vi "Get_Rise_Fall_Time.vi"(10 "Transition_Points":i32[](array[numeric]), 11 "dt":dbl) -> (2 "Fall_Time (s)":dbl, 3 "Rise_Time (s)":dbl)   [LabVIEW 2023]
doc: "This VI Get the rise and fall time when transition points and dt were given in."
uses:
  <vilib>/gmath/NI_Gmath.lvlib
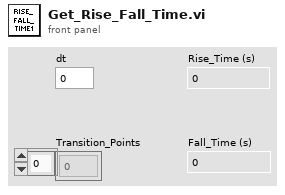
[diagram p1: front panel]
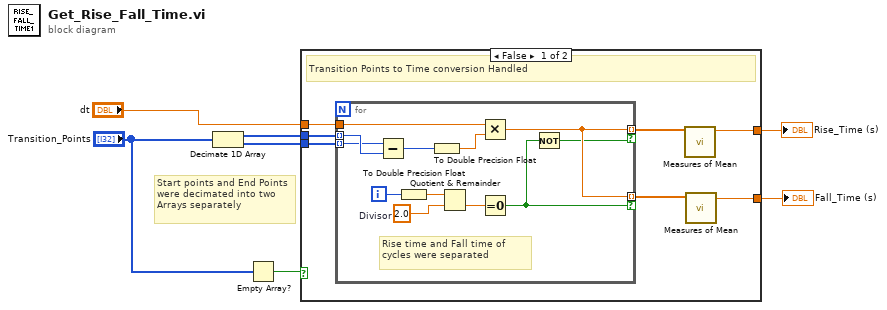
[diagram p0: block diagram]
diagram:
  # "Start points and End Points were decimated into two Arrays separately"
  n1 = Decimate 1D Array("Transition_Points") -> (w3:i32[], w4:i32[])
  n2 = Empty Array?(array="Transition_Points") -> (empty?=w1:bool)
  n3 = case shown="False" w1 {
    tunnel: [w14 _] -> w7
    tunnel: [w12 _] -> w6
    tunnel: "dt" -> [w10 _]
    tunnel: w4 -> [w9 _]
    tunnel: w3 -> [w8 _]
    frame False {
      # "Transition Points to Time conversion Handled"
      n4 = for {
        tunnel: w8 -> [w26] mode=indexing
        tunnel: w9 -> [w25] mode=indexing
        tunnel: w10 -> [w24]
        tunnel: [w21] -> w11 mode=indexing if=w16
        tunnel: [w21] -> w13 mode=indexing if=w17
        i -> [w20]
        w19 = 2.0  # Divisor
        # "Rise time and Fall time of cycles were separated"
        n5 = Subtract(x=w25, y=w26) -> (x-y=w23:i32)
        n6 = To Double Precision Float(number=w20) -> (double precision float=w15:dbl)
        n7 = To Double Precision Float(number=w23) -> (double precision float=w22:dbl)
        n8 = Quotient & Remainder(x=w15, y=w19) -> (floor(x/y)=w18:dbl)  [unwired: 1 out]
        n9 = Multiply(x=w24, y=w22) -> (x*y=w21:dbl)
        n10 = Equal To 0?(x=w18) -> (x = 0?=w17:bool)
        n11 = Not(x=w17) -> (.not. x?=w16:bool)
      }
      n12 = call <vilib>:"Measures of Mean.vi"("x array"=w11) -> ("mean value"=w12:dbl)  [unwired: 9 in, 1 out]
      n13 = call <vilib>:"Measures of Mean.vi"("x array"=w13) -> ("mean value"=w14:dbl)  [unwired: 9 in, 1 out]
    }
    frame True {
      # "No transition Points Condition handled"
    }
  }
  "Rise_Time (s)" <- w6
  "Fall_Time (s)" <- w7
